vi "Check Admin Identity.vi"(8 "error in (no error)":errorcluster, 10 "UserName(\"\")":string, 11 "Member_Actor in":refnum<class "Member_Actor.lvclass">) -> (0 "error out":errorcluster, 2 "CheckIdentity （False）":bool, 3 "Member_Actor out":refnum<class "Member_Actor.lvclass">)   [LabVIEW 2015, in "Member_Actor.lvlib" / "Member_Actor.lvclass"]
uses:
  Member_Actor.lvclass
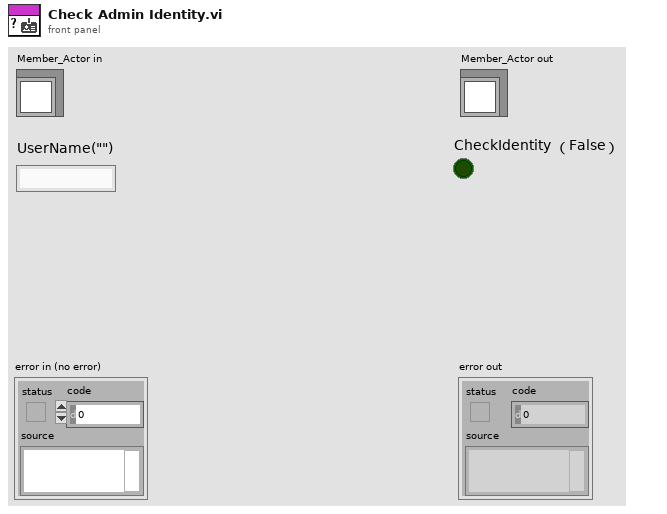
[diagram p1: front panel]
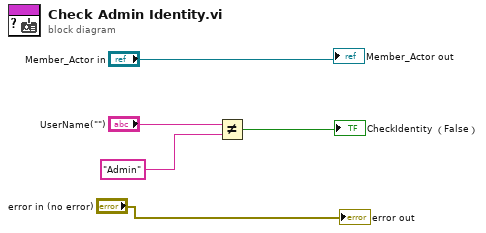
[diagram p0: block diagram]
diagram:
  n1 = Not Equal?(x="UserName(\"\")", y="Admin") -> (x != y?=→"CheckIdentity （False）":bool)
  "error out" <- "error in (no error)"
  "Member_Actor out" <- "Member_Actor in"
